vi "SRV_Search Complete 1D Array(abc).vi"(1 "Start Index (0)":i32, 2 "Element":string, 3 "1D Array":string[](array[string])) -> (0 "Indices Of Elements":i32[](array[numeric]))   [LabVIEW 2009]
doc: "Searches for Element in 1D Array starting at Start Index. Start Index defaults to 0 if unwired. Output is an empty array if function does not find Element.\n\n\nAuthor: Mike Schultz\n\n\nLogicPD, Inc\nwww.logicpd.com"
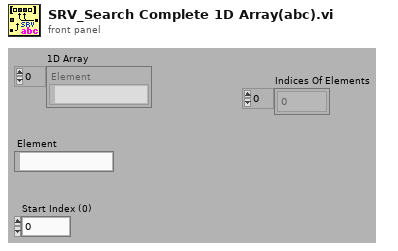
[diagram p1: front panel]
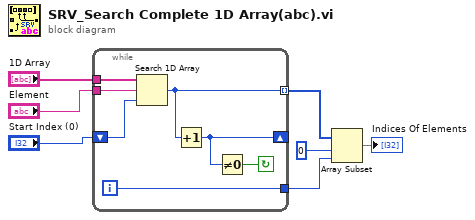
[diagram p0: block diagram]
diagram:
  n1 = while {
    tunnel: [w8] -> w2
    tunnel: [w12] -> w4 mode=indexing
    shift-left: "Start Index (0)" -> [w11]
    shift-right: [w10] -> _
    tunnel: "Element" -> [w13]
    tunnel: "1D Array" -> [w14]
    i -> [w8]
    stop <- w9 continue-if-true
    n2 = Search 1D Array(1D array=w14, element=w13, start index (0)=w11) -> (index of element=w12:i32)
    n3 = Increment(x=w12) -> (x+1=w10:i32)
    n4 = Not Equal To 0?(x=w10) -> (x != 0?=w9:bool)
  }
  n5 = Array Subset(array=w4, index=0, length=w2) -> (→"Indices Of Elements":i32[])
